vi "Next Stock Design.vi"() -> ()   [LabVIEW 2011]
uses:
  Design Server.lvlib
  Folders.ctl
panel:
  out "Stock file names":string[][](array[string])
  in  "versions":i32[](array[numeric])=[-1, 5116, -1, 5125, -1, 5131, -1, -1]
  in  "Methods":string[](array[string])=["EtFlocSedFiLow", "EtFlocSedFi", "Flocculator", "SedTank", "SRSF", "LFOM", "Cdc", "Box"]
  # "This code checks latest master method for SVN version to use for each method\nThen it checks all the method files to see what stock designs are required\nThen it checks the produced design folders to see what has actually been produced.\nIt calculates the number of designs pending\nIt produces one request if there are pending requests"
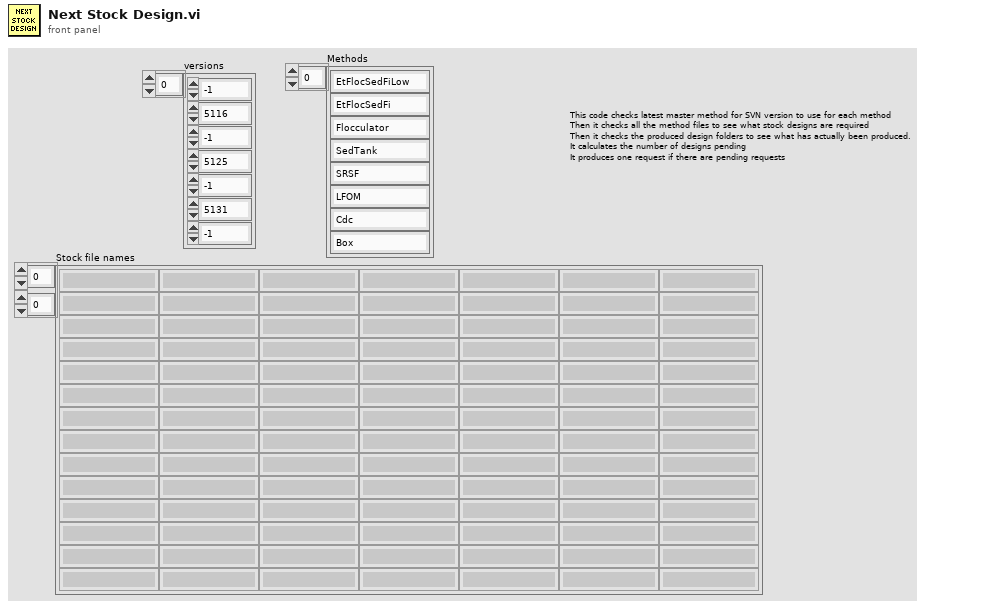
[diagram p1: front panel]
types:
  T1 = typedef "Design Server.lvlib/Folders.ctl" = enum16{"MathcadMethods", "RequestedDesigns", "CompletedDesigns", "MathcadCode", "CollabnetSVN.exe"}
  T2 = typedef "Method.ctl" = cluster{"Title":string, "Rank":string, "About":string, "Input Parameters":cluster{"Description":string, "Name":string, "Min":string, "Max":string, "Default":string, "Units":string, "Increment":string, "Stock designs":string[]}[], "AutoCAD drawings":cluster{"File Name":string, "AC Variables":string[]}[], "Stock file names":string[]}
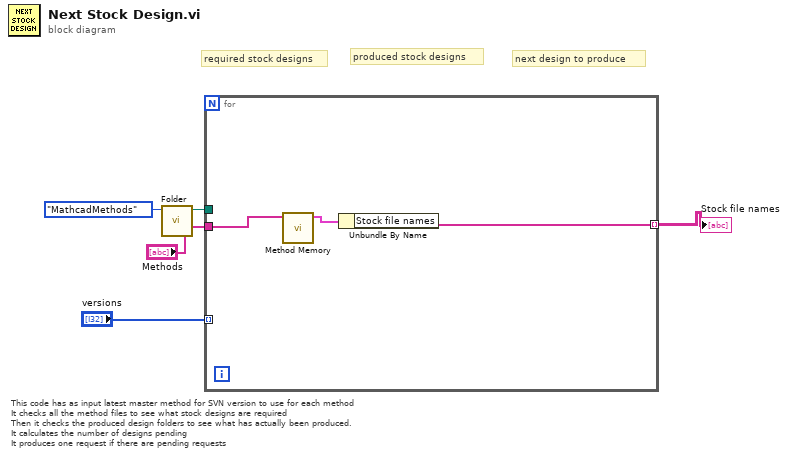
[diagram p0: block diagram]
diagram:
  # "next design to produce"
  # "produced stock designs"
  # "required stock designs"
  # "This code has as input latest master method for SVN version to use for each method\nIt checks all the method files to see what stock designs are required\nThen it checks the produced design folders to see what has actually been produced.\nIt calculates the number of designs pending\nIt produces one request if there are pending requests"
  n1 = call "Folder.vi"("Folders"=Folders."MathcadMethods") -> ("FolderPath"=w4:path)  [unwired: 8 in, 2 out]
  n2 = for {
    tunnel: w4 -> [_]
    tunnel: "Methods" -> [w8]
    tunnel: "versions" -> [_] mode=indexing
    tunnel: [w6] -> w1 mode=indexing
    n3 = call "Method Memory.vi"("Method Name"=w8) -> ("Method Out"=w7:T2)  [unwired: 8 in, 2 out]
    n4 = Unbundle By Name(w7) -> ("Stock file names"=w6:string[])
  }
  "Stock file names" <- w1
